vi "UV-VIS SetReadModeSD.vi"(3 "error in (no error)":errorcluster, 4 "mode":T1, 5 "Control in":refnum<class "CCD_camera.lvclass">) -> (0 "error out":errorcluster, 1 "DLL error code":u32, 2 "Control out":refnum<class "CCD_camera.lvclass">)   [LabVIEW 2018, in "CCD_camera.lvclass"]
doc: "This function will set the readout mode to be used on the subsequent acquisitions.\n\n<B>Parameter:</B>\nmode - readout mode\n Valid values: 0 - Full Vertical Binning\n 1 - Multi-Track\n 2 - Random-Track\n 3 - Single-Track\n 4 - Image\n\n<B>Error codes:</B>\nDRV_SUCCESS - Readout mode set.\nDRV_NOT_INITIALIZED - System not initialized.\nDRV_ACQUIRING - Acquisition in progress.\nDRV_P1INVALID - Invalid readout mode passed."
uses:
  CCD_camera.lvclass
  atmcd32d.llb/ReadMode_mode typedef.ctl
  C:/Users/Sergey Denisov/Documents/REPS/TRANCON/Classes/Detector/Detector.lvclass
  Detector.lvclass/Detector.ctl
  Detector.lvclass
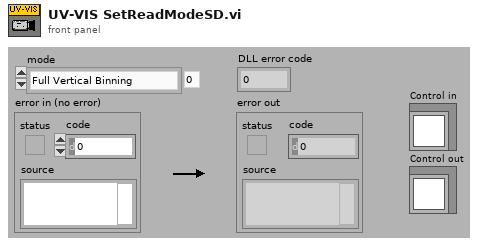
[diagram p1: front panel]
types:
  T1 = typedef "ReadMode_mode typedef.ctl" = enum16{"Full Vertical Binning", "Multi-Track", "Random-Track", "Single-Track", "Image"}
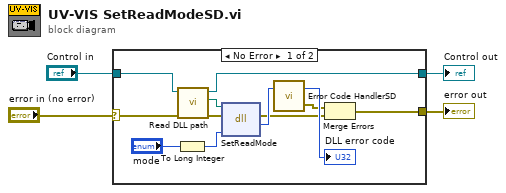
[diagram p0: block diagram]
diagram:
  n1 = case shown="No Error" "error in (no error)" {
    selector: "error in (no error)" -> [w11 w18]
    tunnel: [w6 w18] -> w3
    tunnel: [w5 w17] -> w2
    tunnel: "Control in" -> [w12 w17]
    frame No Error {
      n2 = To Long Integer(number="mode") -> (32bit integer=w14:i32)
      n3 = call "Read DLL path.vi"("error in (no error)"=w11, "Detector in"=w12) -> ("error out"=w10:errorcluster, "DLL path"=w9:path, "Detector out"=w5:refnum<class "CCD_camera.lvclass">)  [unwired: 7 in]
      n4 = dll-call lib="S:/TRANCON/DLL/Atmcd32d.dll" fn="SetReadMode"(path in=w9, error in=w10, "mode"=w14) -> (error out=w8:errorcluster, "return type"=w16:u32)  [unwired: 2 in, 1 out]
      n5 = call "Error Code HandlerSD.vi"("DLL error code"=w16) -> ("error out"=w7:errorcluster, "dup DLL error code"=→"DLL error code":u32)  [unwired: 1 in]
      n6 = Merge Errors(w7, w8) -> (w6:errorcluster)
    }
    frame Error {
    }
  }
  "error out" <- w3
  "Control out" <- w2
